vi "move_1.vi"() -> (0 "Enum":T1(ring))   [LabVIEW 2016]
uses:
  <vilib>/NXT/Block Support/NXT_OutputPort.ctl
  <vilib>/NXT/NXTIO Xnodes/NXTIONodeSubVIs/NXTStopMotors.vi
  <vilib>/NXT/NXTIO Xnodes/NXTIONodeSubVIs/NXTMotorRunDistance.vi
  <vilib>/NXT/NXTIO Xnodes/NXTIONodeSubVIs/LEGOMotorStatus.vi
  <vilib>/NXT/NXTIO Xnodes/NXTIONodeSubVIs/NXTMoveMotors.vi
  <vilib>/NXT/NXTIO Xnodes/NXTIONodeSubVIs/LEGOResetMotors.vi
  <vilib>/NXT/NXTIO Xnodes/AddressXNode/NXTIOAddress.xnode
  <vilib>/NXT/Subs/LVHSConnector.ctl
  <vilib>/NXT/NXTIO Xnodes/NXTIOXNode/NXTIO.xnode
  <vilib>/NXT/LegoClasses/BrickReference/BrickReference.lvclass
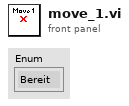
[diagram p1: front panel]
types:
  T1 = enum16{"Bereit", "Move 1", "Reference_pos", "Wait", "row1_check", "row2_check", "row3_check", "return", "move2", "move3", "move4", "move5", "end"}
  T2 = enum16{"forward", "mark", "pause", "up", "return", "end"}
  T3 = typedef "NXT_OutputPort.ctl" = u8
  T4 = cluster{"Output Port":T3, "Output Port 2":T3, "Output Port 3":T3}
  T5 = typedef "LVHSConnector.ctl" = refnum<class "BrickReference.lvclass">
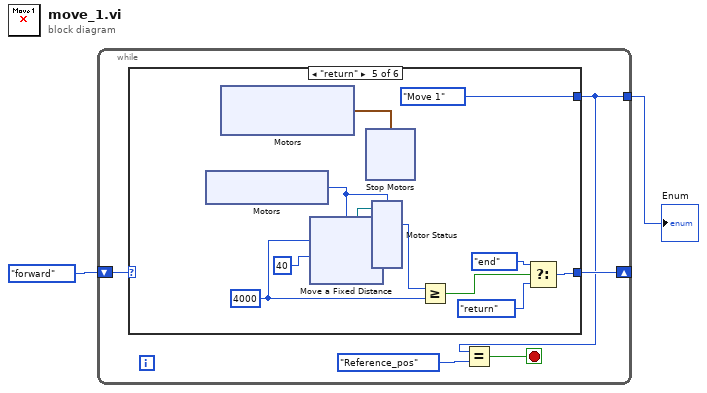
[diagram p0: block diagram]
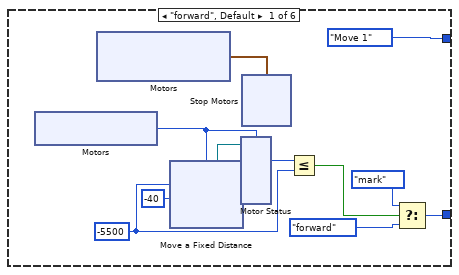
[diagram p2: hidden frame]
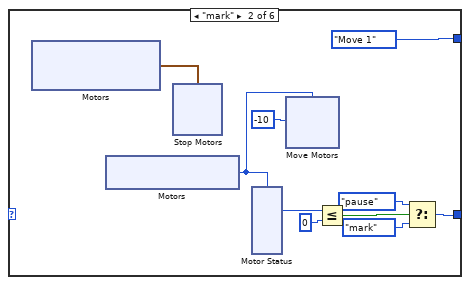
[diagram p3: hidden frame]
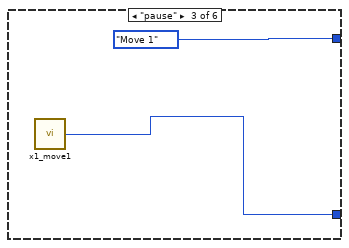
[diagram p4: hidden frame]
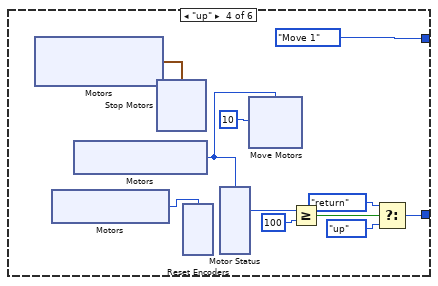
[diagram p5: hidden frame]
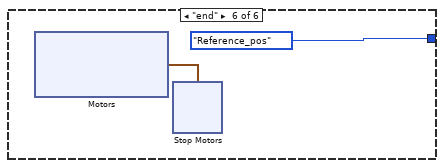
[diagram p6: hidden frame]
diagram:
  n1 = while {
    shift-right: [w7] -> _
    shift-left: T2."forward" -> [w6]
    tunnel: [w5] -> w2
    stop <- w4 stop-if-true
    n2 = case shown="\"return\"" w6 {
      tunnel: [w10 w51 w76 w85 w118 _] -> w7
      tunnel: [T1."Move 1" T1."Move 1" T1."Move 1" T1."Move 1" T1."Move 1" T1."Reference_pos"] -> w5
      frame "forward", Default {
        w14 = -5500 ("Distance 1")
        n3 = xnode "Motors"() -> ("Motor"=w9:T3)
        n4 = xnode "Motors"() -> ("Motor"=w18:cluster{"Port":T3, "Port":T3})
        n5 = xnode "Move a Fixed Distance"("Speed 1"=i8 -40, "Distance 1"=w14, "Motors"=w9) -> ("NXT/EV3"=w8:T5)  [unwired: 1 in]
        n6 = xnode "Motor Status"("Motors"=w9, "NXT/EV3"=w8) -> ("Position 1"=w15:i32)  [unwired: 2 out]
        n7 = xnode "Stop Motors"("Motors"=w18) -> ()  [unwired: 1 in, 1 out]
        n8 = Less Or Equal?(x=w15, y=w14) -> (x <= y?=w12:bool)
        n9 = Select(t=T2."mark", s=w12, f=T2."forward") -> (s? t:f=w10:T2)
      }
      frame "mark" {
        n10 = xnode "Motors"() -> ("Motor"=w53:cluster{"Port":T3, "Port":T3})
        n11 = xnode "Motors"() -> ("Motor"=w48:T3)
        n12 = xnode "Stop Motors"("Motors"=w53) -> ()  [unwired: 1 in, 1 out]
        n13 = xnode "Motor Status"("Motors"=w48) -> ("Position 1"=w47:i32)  [unwired: 1 in, 2 out]
        n14 = xnode "Move Motors"("Power/Speed 1"=i8 -10, "Motors"=w48) -> ()  [unwired: 1 in, 1 out]
        n15 = Less Or Equal?(x=w47, y=0) -> (x <= y?=w45:bool)
        n16 = Select(t=T2."pause", s=w45, f=T2."mark") -> (s? t:f=w51:T2)
      }
      frame "pause" {
        n17 = call "x1_move1.vi"() -> ("Enum"=w76:T2)  [unwired: 1 in]
      }
      frame "up" {
        n18 = xnode "Motors"() -> ("Motor"=w87:cluster{"Port":T3, "Port":T3})
        n19 = xnode "Motors"() -> ("Motor"=w78:T3)
        n20 = xnode "Motors"() -> ("Motor"=w81:T3)
        n21 = xnode "Stop Motors"("Motors"=w87) -> ()  [unwired: 1 in, 1 out]
        n22 = xnode "Reset Encoders"("Motors"=w78) -> ()  [unwired: 1 in, 1 out]
        n23 = xnode "Motor Status"("Motors"=w81) -> ("Position 1"=w82:i32)  [unwired: 1 in, 2 out]
        n24 = xnode "Move Motors"("Power/Speed 1"=i8 10, "Motors"=w81) -> ()  [unwired: 1 in, 1 out]
        n25 = Greater Or Equal?(x=w82, y=100) -> (x >= y?=w86:bool)
        n26 = Select(t=T2."return", s=w86, f=T2."up") -> (s? t:f=w85:T2)
      }
      frame "return" {
        w121 = 4000 ("Distance 1")
        n27 = xnode "Motors"() -> ("Motor"=w117:T3)
        n28 = xnode "Motors"() -> ("Motor"=w126:cluster{"Port":T3, "Port":T3})
        n29 = xnode "Move a Fixed Distance"("Speed 1"=i8 40, "Distance 1"=w121, "Motors"=w117) -> ("NXT/EV3"=w116:T5)  [unwired: 1 in]
        n30 = xnode "Stop Motors"("Motors"=w126) -> ()  [unwired: 1 in, 1 out]
        n31 = xnode "Motor Status"("Motors"=w117, "NXT/EV3"=w116) -> ("Position 1"=w123:i32)  [unwired: 2 out]
        n32 = Greater Or Equal?(x=w123, y=w121) -> (x >= y?=w120:bool)
        n33 = Select(t=T2."end", s=w120, f=T2."return") -> (s? t:f=w118:T2)
      }
      frame "end" {
        n34 = xnode "Motors"() -> ("Motor"=w153:cluster{"Port":T3, "Port":T3, "Port":T3})
        n35 = xnode "Stop Motors"("Motors"=w153) -> ()  [unwired: 1 in, 1 out]
      }
    }
    n36 = Equal?(x=w5, y=T1."Reference_pos") -> (x = y?=w4:bool)
  }
  "Enum" <- w2
